vi "LoadAWG.vi"(8 "error in":errorcluster, 11 "file (use dialog)":path) -> (0 "error out":errorcluster, 2 "dt(s)":dbl, 3 "AWGs":dbl[][](array[numeric]))   [LabVIEW 2018]
uses:
  <vilib>/Utility/file.llb/Read Delimited Spreadsheet (DBL).vi
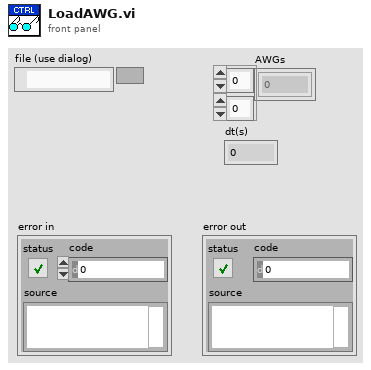
[diagram p1: front panel]
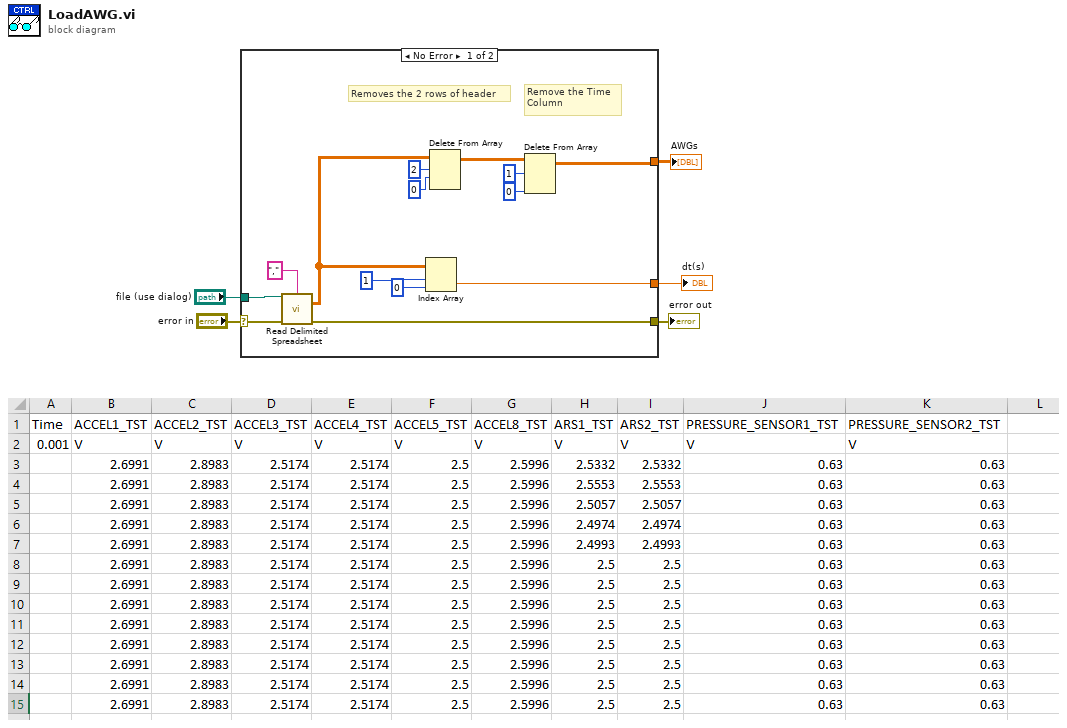
[diagram p0: block diagram]
diagram:
  n1 = case shown="No Error" "error in" {
    selector: "error in" -> [w17 w20]
    tunnel: [w15 w20] -> w5
    tunnel: [w7 _] -> w3
    tunnel: [w11 _] -> w2
    tunnel: "file (use dialog)" -> [w16 _]
    frame No Error {
      # "Remove the Time\nColumn"
      # "Removes the 2 rows of header"
      n2 = call-poly <vilib>:"Read Delimited Spreadsheet.vi"("file path (dialog if empty)"=w16, "error in (no error)"=w17, "delimiter (\\t)"="," ("delimiter (\\t)")) -> ("all rows"=w14:dbl[][], "error out"=w15:errorcluster)  [unwired: 7 in, 4 out]
      n3 = Index Array(array=w14, index (row)=1, index (col)=0 ("disabled index (col)")) -> (element=w11:dbl)
      n4 = Delete From Array(array=w14, length=2, index (row)=0) -> (array with subset deleted=w10:dbl[][])  [unwired: 1 in, 1 out]
      n5 = Delete From Array(array=w10, length=1, index (col)=0 ("disabled index (col)")) -> (array with subset deleted=w7:dbl[][])  [unwired: 1 in, 1 out]
    }
    frame Error {
    }
  }
  "error out" <- w5
  "AWGs" <- w3
  "dt(s)" <- w2
